vi "boolean array to string.vi"(4 "Boolean array Input":bool[](array[boolean])) -> (1 "String Output":string)   [LabVIEW 2020]
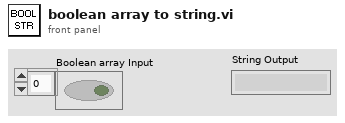
[diagram p1: front panel]
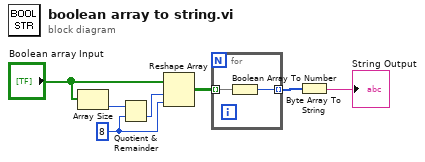
[diagram p0: block diagram]
diagram:
  w6 = 8 ("dimension size")
  n1 = Array Size(array="Boolean array Input") -> (size(s)=w3:i32)
  n2 = Quotient & Remainder(x=w3, y=w6) -> (floor(x/y)=w5:i32)  [unwired: 1 out]
  n3 = Reshape Array("Boolean array Input", w5, w6) -> (w4:bool[][])
  n4 = for {
    tunnel: w4 -> [w9] mode=indexing
    tunnel: [w8] -> w1 mode=indexing
    n5 = Boolean Array To Number(Boolean array=w9) -> (number=w8:u8)
  }
  n6 = Byte Array To String(unsigned byte array=w1) -> (string=→"String Output":string)
